vi "StringFromToDateTimeConvertToMinute.vi"(9 "FromToTime":string="06:21:27 to 09:57:02", 11 "FromToDate":string="31-12-14 to 31-12-14") -> (0 "Min":dbl, 1 "End":string, 3 "Start":string, 4 "EndMDY":string, 5 "StartMDY":string)   [LabVIEW 2012]
uses:
  <vilib>/Utility/miscctls.llb/LVDateTimeRec.ctl
panel:
  out "x-y":dbl
  in  "date time rec":T1
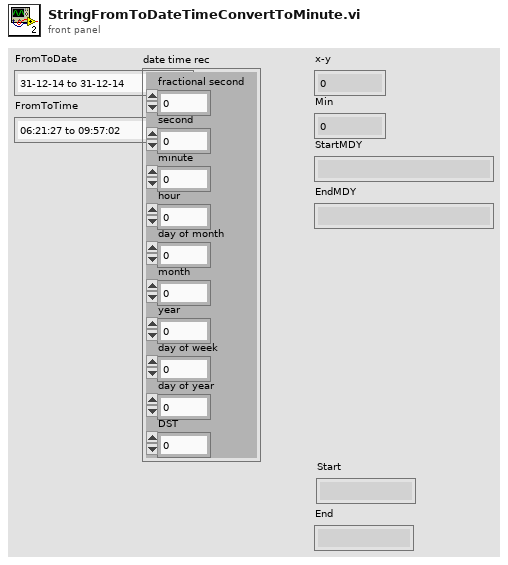
[diagram p1: front panel]
types:
  T1 = typedef "LVDateTimeRec.ctl" = cluster{"fractional second":dbl, "second":i32, "minute":i32, "hour":i32, "day of month":i32, "month":i32, "year":i32, "day of week":i32, "day of year":i32, "DST":i32}
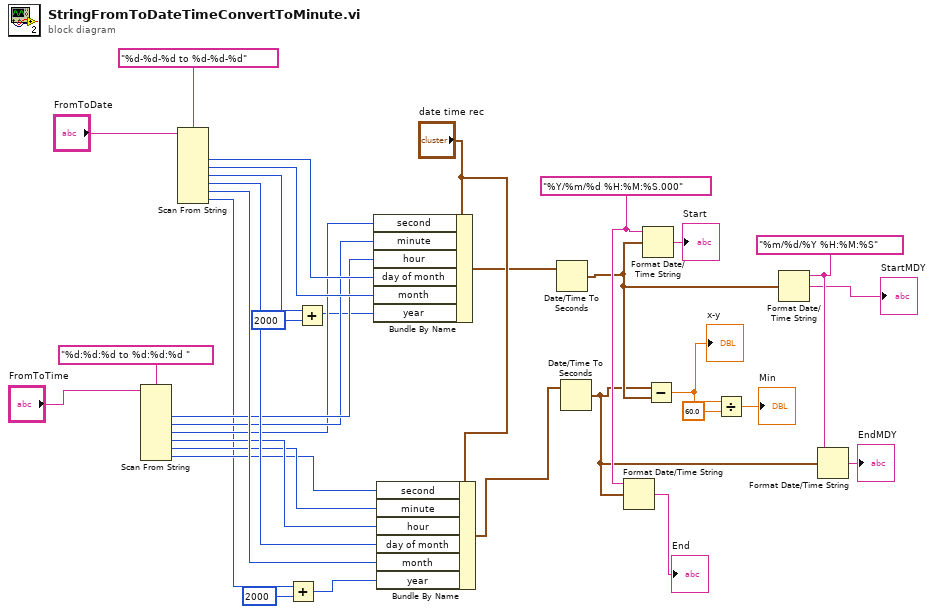
[diagram p0: block diagram]
diagram:
  w3 = "%m/%d/%Y %H:%M:%S" ("time format string (%c)")
  w8 = "%Y/%m/%d %H:%M:%S.000" ("time format string (%c)")
  n1 = Scan From String(format string="%d:%d:%d to %d:%d:%d ", input string="FromToTime") -> (output 1=w25:i32, output 2=w24:i32, output 3=w23:i32, output 4=w22:i32, output 5=w21:i32, output 6=w20:i32)  [unwired: 8 in, 3 out]
  n2 = Scan From String(format string="%d-%d-%d to %d-%d-%d", input string="FromToDate") -> (output 1=w30:i32, output 2=w29:i32, output 3=w19:i32, output 4=w27:i32, output 5=w26:i32, output 6=w15:i32)  [unwired: 8 in, 3 out]
  n3 = Add(x=w15, y=2000) -> (x+y=w14:i32)
  n4 = Add(x=w19, y=2000) -> (x+y=w18:i32)
  n5 = Bundle By Name(cluster="date time rec", "second"=w23, "minute"=w24, "hour"=w25, "day of month"=w30, "month"=w29, "year"=w18) -> (w13:T1)
  n6 = Bundle By Name(cluster="date time rec", "second"=w20, "minute"=w21, "hour"=w22, "day of month"=w27, "month"=w26, "year"=w14) -> (w12:T1)
  n7 = Date/Time To Seconds(2:w13) -> (0:w5:timestamp)  [unwired: 1 in]
  n8 = Date/Time To Seconds(2:w12) -> (0:w4:timestamp)  [unwired: 1 in]
  n9 = Format Date/Time String(time format string (%c)=w8, seconds (now)=w4) -> (date/time string=→"End":string)  [unwired: 1 in]
  n10 = Format Date/Time String(time format string (%c)=w8, seconds (now)=w5) -> (date/time string=→"Start":string)  [unwired: 1 in]
  n11 = Subtract(x=w4, y=w5) -> (x-y=w11:dbl)
  "x-y" <- w11
  n12 = Divide(x=w11, y=60.0) -> (x/y=→"Min":dbl)
  n13 = Format Date/Time String(time format string (%c)=w3, seconds (now)=w5) -> (date/time string=→"StartMDY":string)  [unwired: 1 in]
  n14 = Format Date/Time String(time format string (%c)=w3, seconds (now)=w4) -> (date/time string=→"EndMDY":string)  [unwired: 1 in]
